vi "DCLeft.vi"(11 "Dc In":dbl) -> (3 "PWM Left Motor":T1={"period (uSec)"=20000, "pulse width (uSec)"=1500})   [LabVIEW 2016]
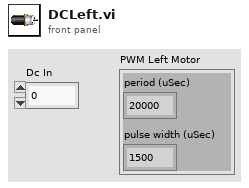
[diagram p1: front panel]
types:
  T1 = cluster{"period (uSec)":u32, "pulse width (uSec)":u32}
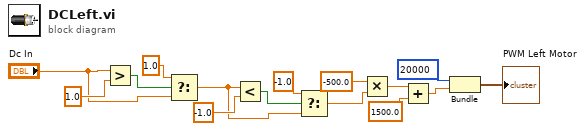
[diagram p0: block diagram]
diagram:
  n1 = Greater?(x="Dc In", y=1.0) -> (0:w14:bool)
  n2 = Select(t=1.0, s=w14, f="Dc In") -> (s? t:f=w9:dbl)
  n3 = Less?(x=w9, y=-1.0) -> (x < y?=w11:bool)
  n4 = Select(t=-1.0, s=w11, f=w9) -> (s? t:f=w5:dbl)
  n5 = Multiply(x=-500.0, y=w5) -> (x*y=w4:dbl)
  n6 = Add(x=w4, y=1500.0) -> (x+y=w2:dbl)
  n7 = Bundle(20000, w2) -> (→"PWM Left Motor":cluster{i32, dbl})  [unwired: 1 in]
